vi "Get Auto Mode from arrays.vi"(9 "Auto Name":string, 10 "Programs":string[](array[string]), 11 "Program Name":string[](array[string])) -> (2 "index":i32, 3 "Auto Program":string)   [LabVIEW 2013]
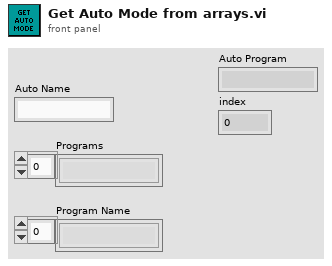
[diagram p1: front panel]
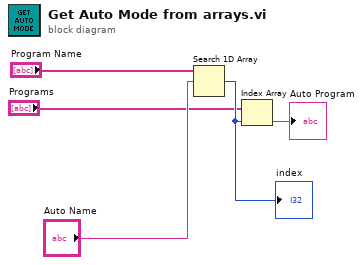
[diagram p0: block diagram]
diagram:
  n1 = Search 1D Array(1D array="Program Name", element="Auto Name") -> (index of element=w3:i32)  [unwired: 1 in]
  "index" <- w3
  n2 = Index Array(array="Programs", index=w3) -> (element=→"Auto Program":string)
